vi "Manually Remove Actor.vi"(8 "error in (no error)":errorcluster, 10 "Actor's Q":refnum<class "Message Enqueuer.lvclass">, 11 "Actor Monitor New in":refnum<class "Actor Monitor.lvclass">) -> (0 "error out":errorcluster, 3 "Actor Monitor New out":refnum<class "Actor Monitor.lvclass">)   [LabVIEW 2020, in "Monitored Actor.lvlib" / "Actor Monitor.lvclass"]
doc: "Removes the actor from the monitoring list\n\nCopyright: MGI 2016\nAuthor: Derek Trepanier"
uses:
  <vilib>/MGI/Monitored Actor/Actor Monitor/Actor Monitor/Actor Monitor.lvclass
  <vilib>/ActorFramework/Message Enqueuer/Message Enqueuer.lvclass
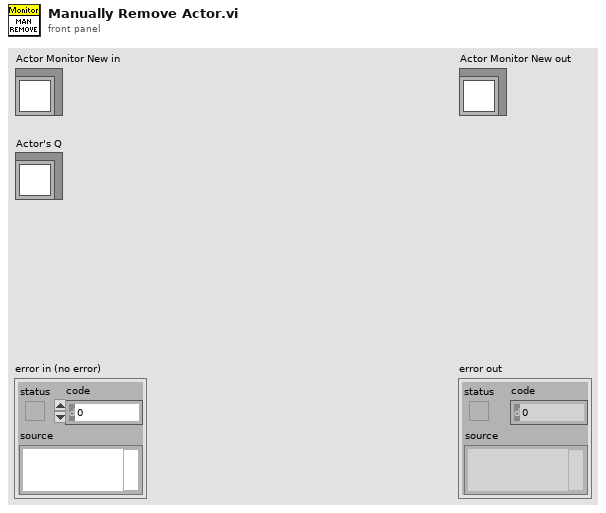
[diagram p1: front panel]
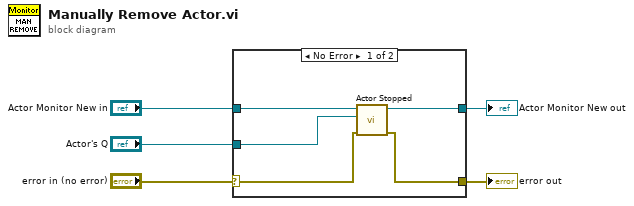
[diagram p0: block diagram]
diagram:
  n1 = case shown="No Error" "error in (no error)" {
    selector: "error in (no error)" -> [w7 w12]
    tunnel: [w6 w12] -> w4
    tunnel: [w9 w11] -> w2
    tunnel: "Actor Monitor New in" -> [w10 w11]
    tunnel: "Actor's Q" -> [w8 _]
    frame No Error {
      n2 = call <vilib>:"Actor Stopped.vi"("error in (no error)"=w7, "Actor's Self Q"=w8, "Actor Monitor New in"=w10) -> ("error out"=w6:errorcluster, "Actor Monitor New out"=w9:refnum<class "Actor Monitor.lvclass">)  [unwired: 7 in]
    }
    frame Error {
    }
  }
  "error out" <- w4
  "Actor Monitor New out" <- w2
